vi "RunOperation.vi"(10 "Inputs":string[](array[string]), 11 "LUnitCLI In":refnum<class "LUnitCLI.lvclass">) -> (1 "Output/Failure":string, 2 "CLI Process Return Code":i32, 3 "LUnitCLI Out":refnum<class "LUnitCLI.lvclass">)   [LabVIEW 2020, in "LUnitCLI.lvclass"]
uses:
  LUnitCLI.lvclass
  LUnitCLI.lvclass/LUnitCLI.ctl
  User Interface/Execution API/Execution API.lvclass
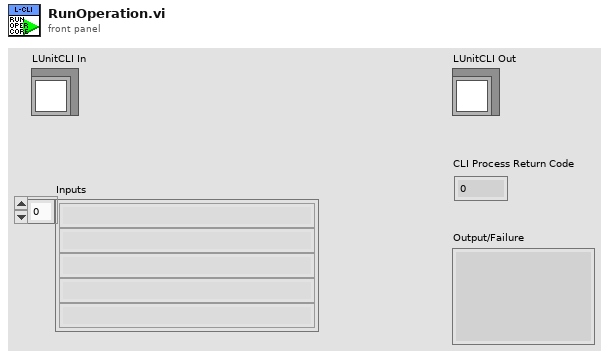
[diagram p1: front panel]
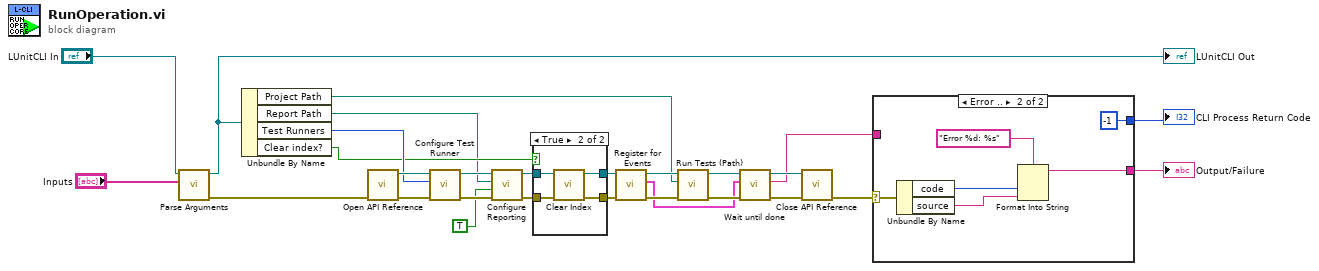
[diagram p0: block diagram]
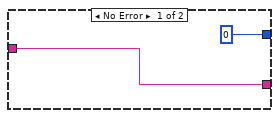
[diagram p3: hidden frame]
diagram:
  n1 = call "Parse Arguments.vi"("Inputs"="Inputs", "LUnitCLI In"="LUnitCLI In") -> ("error out"=w4:errorcluster, "LUnitCLI Out"=w24:refnum<class "LUnitCLI.lvclass">)  [unwired: 8 in]
  "LUnitCLI Out" <- w24
  n2 = Unbundle By Name(w24) -> ("Project Path"=w2:path, "Report Path"=w7:path, "Test Runners"=w9:i32, "Clear index?"=w8:bool)
  n3 = call "Open API Reference.vi"("error in (no error)"=w4) -> ("error out"=w22:errorcluster, "Execution API out"=w23:refnum<class "Execution API.lvclass">)  [unwired: 9 in]
  n4 = call "Configure Test Runner.vi"("error in (no error)"=w22, "Number of Test Runners"=w9, "Execution API In"=w23) -> ("error out"=w20:errorcluster, "Execution API Out"=w21:refnum<class "Execution API.lvclass">)  [unwired: 7 in]
  n5 = call "Configure Reporting.vi"("error in (no error)"=w20, "Autogenerate?"=TRUE, "Path"=w7, "Execution API In"=w21) -> ("error out"=w18:errorcluster, "Execution API Out"=w19:refnum<class "Execution API.lvclass">)  [unwired: 6 in]
  n6 = case shown="True" w8 {
    tunnel: w19 -> [w30 w34]
    tunnel: w18 -> [w29 w33]
    tunnel: [w30 w32] -> w17
    tunnel: [w29 w31] -> w16
    frame False {
    }
    frame True {
      n7 = call "Clear Index.vi"("error in (no error)"=w33, "Execution API In"=w34) -> ("error out"=w31:errorcluster, "Execution API Out"=w32:refnum<class "Execution API.lvclass">)  [unwired: 8 in]
    }
  }
  n8 = call "Register for Events.vi"("error in (no error)"=w16, "Execution API in"=w17) -> ("error out"=w14:errorcluster, "Event Registrations"=w1:cluster{"placeholder":bool}, "Execution API out"=w15:refnum<class "Execution API.lvclass">)  [unwired: 7 in]
  n9 = call "Run Tests (Path).vi"("error in (no error)"=w14, "Project or Class Path"=w2, "Execution API In"=w15) -> ("error out"=w12:errorcluster, "Execution API Out"=w13:refnum<class "Execution API.lvclass">)  [unwired: 7 in]
  n10 = call "Wait until done.vi"("error in (no error)"=w12, "Result Registration Refnum"=w1, "Execution API In"=w13) -> ("error out"=w10:errorcluster, "Output"=w5:string, "Execution API Out"=w11:refnum<class "Execution API.lvclass">)  [unwired: 6 in]
  n11 = call "Close API Reference.vi"("error in (no error)"=w10, "Execution API in"=w11) -> ("error out"=w3:errorcluster)  [unwired: 9 in]
  n12 = case shown="Error .." w3 {
    selector: w3 -> [_ w41]
    tunnel: [w36 w37] -> w28
    tunnel: w5 -> [w36 _]
    tunnel: [0 ("CLI Process Return Code") -1 ("CLI Process Return Code")] -> w27
    frame No Error {
    }
    frame Error {
      n13 = Unbundle By Name(w41) -> ("code"=w40:i32, "source"=w39:string)
      n14 = Format Into String(format string="Error %d: %s", w40, w39) -> (resulting string=w37:string)  [unwired: 2 in, 1 out]
    }
  }
  "CLI Process Return Code" <- w27
  "Output/Failure" <- w28
